vi "Untitled 3 (SubVI).vi"(10 "Gyro  Data (dps)":T1, 11 "Acceleration Data (g)":T1) -> (1 "Gyro_X":dbl, 2 "Accel_Z":dbl, 3 "Accel_Y":dbl, 4 "Gyro_Y":dbl, 5 "Accel_X":dbl, 6 "Gyro_Z":dbl)   [LabVIEW 2016]
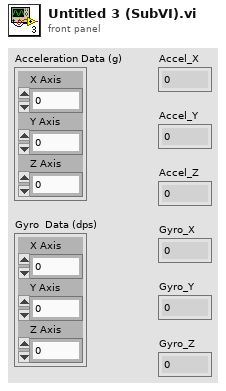
[diagram p1: front panel]
types:
  T1 = cluster{"X Axis":i16, "Y Axis":i16, "Z Axis":i16}
  T2 = cluster{"X Axis":dbl, "Y Axis":dbl, "Z Axis":dbl}
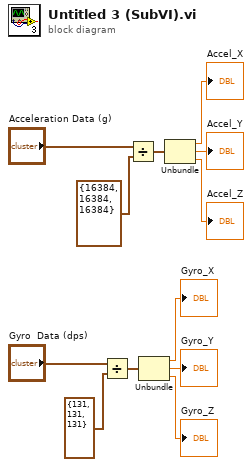
[diagram p0: block diagram]
diagram:
  n1 = Divide(x="Gyro  Data (dps)", y=T1 {"X Axis"=131, "Y Axis"=131, "Z Axis"=131}) -> (x/y=w1:T2)
  n2 = Divide(x="Acceleration Data (g)", y=T1 {"X Axis"=16384, "Y Axis"=16384, "Z Axis"=16384}) -> (x/y=w3:T2)
  n3 = Unbundle(w1) -> ("X Axis"=→"Gyro_X":dbl, "Y Axis"=→"Gyro_Y":dbl, "Z Axis"=→"Gyro_Z":dbl)
  n4 = Unbundle(w3) -> ("X Axis"=→"Accel_X":dbl, "Y Axis"=→"Accel_Y":dbl, "Z Axis"=→"Accel_Z":dbl)
